vi "Lazy Loader.vi"(8 "error in (no error)":errorcluster, 11 "object in":refnum<class "Button.lvclass">) -> (0 "error out":errorcluster, 3 "object out":refnum<class "Button.lvclass">)   [LabVIEW 2012, in "Button.lvclass"]
doc: "Replace the current button with its real implementation if the implementation path is different from the actual current value's path and is not empty."
uses:
  Button.lvclass
  Button.lvclass/Button.ctl
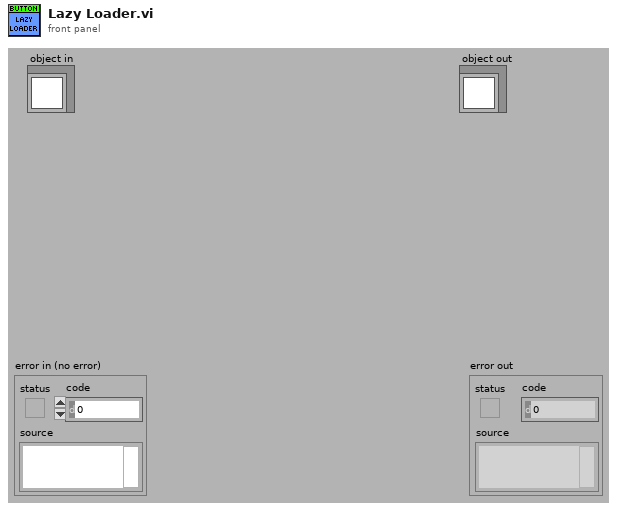
[diagram p1: front panel]
types:
  T1 = typedef "Button.lvclass/Button Type.ctl" = enum16{"Transitory", "Latching"}
  T2 = typedef "Button.lvclass/Button Status.ctl" = enum16{"Off", "Hover", "On", "Disabled"}
  T3 = typedef "imagedata.ctl" = cluster{"image type":i32, "image depth":i32, "image":u8[], "mask":u8[], "colors":u32[], "Rectangle":cluster{"left":i16, "top":i16, "right":i16, "bottom":i16}}
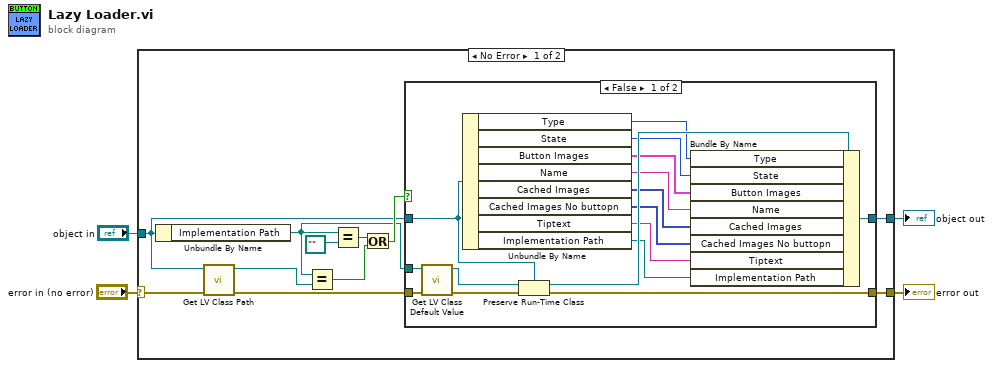
[diagram p0: block diagram]
diagram:
  n1 = case shown="No Error" "error in (no error)" {
    selector: "error in (no error)" -> [w11 w35]
    tunnel: [w7 w35] -> w3
    tunnel: [w9 w34] -> w1
    tunnel: "object in" -> [w8 w34]
    frame No Error {
      n2 = Unbundle By Name(w8) -> ("Implementation Path"=w5:path)
      n3 = call <vilib>:"Get LV Class Path.vi"("error in (no error)"=w11, "object"=w8) -> ("error out"=w6:errorcluster, "class path"=w14:path)  [unwired: 8 in]
      n4 = Equal?(x=w5, y=w14) -> (x = y?=w12:bool)
      n5 = Equal?(x=w5, y=path "") -> (x = y?=w13:bool)
      n6 = Or(x=w13, y=w12) -> (x .or. y?=w10:bool)
      n7 = case shown="False" w10 {
        tunnel: [w24 w33] -> w9
        tunnel: w8 -> [w27 w33]
        tunnel: [w25 w32] -> w7
        tunnel: w6 -> [w30 w32]
        tunnel: w5 -> [w31 _]
        frame False {
          n8 = call <vilib>:"Get LV Class Default Value.vi"("error in (no error)"=w30, "class path"=w31) -> ("error out"=w28:errorcluster, "object"=w29:refnum<class>)  [unwired: 8 in]
          n9 = Unbundle By Name(w27) -> ("Type"=w23:T1, "State"=w22:T2, "Button Images"=w21:T3[], "Name"=w20:string, "Cached Images"=w19:picture[], "Cached Images No buttopn"=w18:picture[], "Tiptext"=w17:string, "Implementation Path"=w16:path)
          n10 = Preserve Run-Time Class(object in=w29, error in=w28, 2:w27) -> (object out=w26:refnum<class "Button.lvclass">, error out=w25:errorcluster)
          n11 = Bundle By Name(cluster=w26, "Type"=w23, "State"=w22, "Button Images"=w21, "Name"=w20, "Cached Images"=w19, "Cached Images No buttopn"=w18, "Tiptext"=w17, "Implementation Path"=w16) -> (w24:refnum<class "Button.lvclass">)
        }
        frame True {
        }
      }
    }
    frame Error {
    }
  }
  "error out" <- w3
  "object out" <- w1
